vi "Create Destroy Discrete Notifier.vi"(6 "Create":bool, 8 "error in":errorcluster, 11 "FPGA-DIO in":refnum<class "FPGA_DIO.lvclass">) -> (0 "error out":errorcluster, 3 "FPGA-DIO out":refnum<class "FPGA_DIO.lvclass">)   [LabVIEW 2019, in "FPGA_DIO.lvlib" / "FPGA_DIO.lvclass"]
uses:
  Library/FPGA_DIO.lvclass
  C:/Users/Public/Documents/Development/builds/Instruments/Instruments.lvlibp/Library/Instruments.lvclass
  Library/FPGA_DIO.lvclass/FPGA_DIO.ctl
  builds/Instruments/Instruments.lvlibp/Accessors/Read Resource.vi
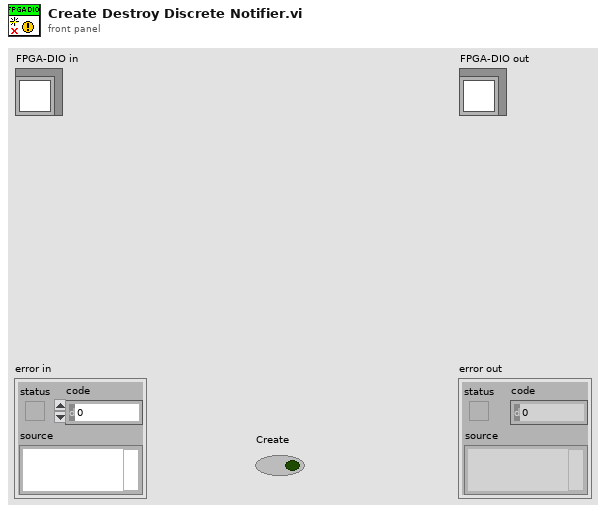
[diagram p1: front panel]
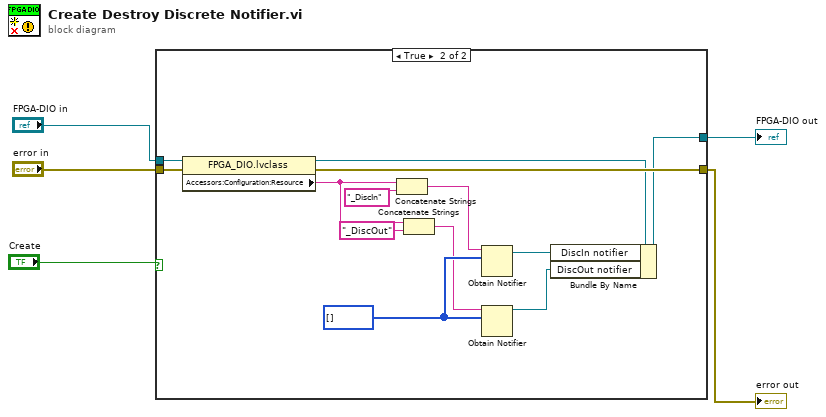
[diagram p0: block diagram]
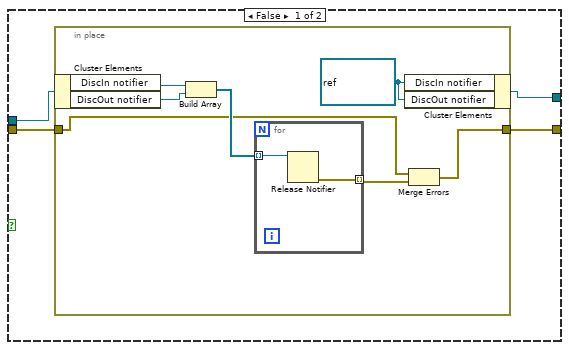
[diagram p2: hidden frame]
diagram:
  n1 = case shown="True" "Create" {
    tunnel: "error in" -> [w8 w31]
    tunnel: [w7 w30] -> w3
    tunnel: "FPGA-DIO in" -> [w9 w29]
    tunnel: [w6 w26] -> w4
    frame False {
      n2 = in-place {
        in-place-border: w8 -> [w11]
        in-place-border: [w10] -> w7
        w16 = refnum<notifier> refnum ("DiscIn notifier")
        n3 = in-place-cluster #1(w9) -> ("DiscIn notifier"=w15:refnum<notifier>, "DiscOut notifier"=w14:refnum<notifier>)
        n4 = Build Array(w15, w14) -> (w13:refnum<notifier>[])
        n5 = for {
          tunnel: w13 -> [w18] mode=indexing
          tunnel: [w17] -> w12 mode=indexing
          n6 = Release Notifier(notifier=w18) -> (error out=w17:errorcluster)  [unwired: 2 in, 2 out]
        }
        n7 = in-place-cluster #1("DiscIn notifier"=w16, "DiscOut notifier"=w16) -> (w6:refnum<class "FPGA_DIO.lvclass">)
        n8 = Merge Errors(w11, w12) -> (w10:errorcluster)
      }
    }
    frame True {
      w27 = u8[] []
      n9 = property class="FPGA_DIO.lvclass"(reference=w29, error in=w31) -> (reference out=w28:refnum<class "FPGA_DIO.lvclass">, error out=w30:errorcluster, "Accessors:Configuration:Resource"=w23:string)
      n10 = Concatenate Strings(w23, "_DiscIn" ("string")) -> (w21:string)
      n11 = Concatenate Strings(w23, "_DiscOut" ("string")) -> (w20:string)
      n12 = Obtain Notifier(name (unnamed)=w21, notification data type=w27) -> (notifier out=w25:refnum<notifier>)  [unwired: 2 in, 2 out]
      n13 = Obtain Notifier(name (unnamed)=w20, notification data type=w27) -> (notifier out=w19:refnum<notifier>)  [unwired: 2 in, 2 out]
      n14 = Bundle By Name(cluster=w28, "DiscIn notifier"=w25, "DiscOut notifier"=w19) -> (w26:refnum<class "FPGA_DIO.lvclass">)
    }
  }
  "error out" <- w3
  "FPGA-DIO out" <- w4
